vi "Boolean to String.vi"(11 "Boolean In":bool) -> (0 "TRUE/FALSE?":string, 1 "1/0":string, 2 "T/F?":string, 3 "ON/OFF?":string, 4 "OK/NOK":string)   [LabVIEW 2020]
doc: "Returns two string depending on the state of the boolean.\n\nEither can be used depending on what type of string is desired."
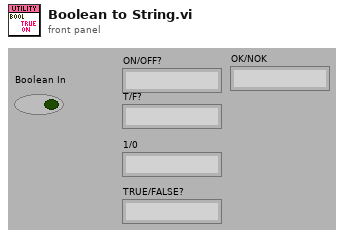
[diagram p1: front panel]
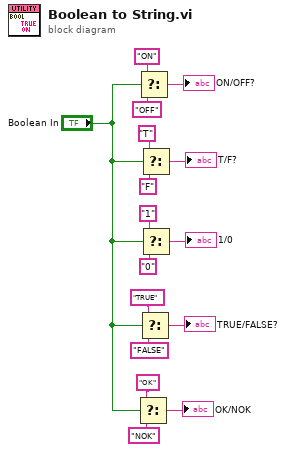
[diagram p0: block diagram]
diagram:
  n1 = Select(t="OK", s="Boolean In", f="NOK") -> (s? t:f=→"OK/NOK":string)
  n2 = Select(t="ON", s="Boolean In", f="OFF") -> (s? t:f=→"ON/OFF?":string)
  n3 = Select(t="TRUE", s="Boolean In", f="FALSE") -> (s? t:f=→"TRUE/FALSE?":string)
  n4 = Select(t="T", s="Boolean In", f="F") -> (s? t:f=→"T/F?":string)
  n5 = Select(t="1", s="Boolean In", f="0") -> (s? t:f=→"1/0":string)
